vi "iterative_thinned_image_to_segment.vi"(3 "1D image array":u8[](array[numeric]), 4 "Segment Start Idx":i32, 5 "Image Height":i32) -> (0 "Algorithm timed out":bool, 1 "Endpoints":i32[](array[numeric]), 2 "Segment Sequence Cluster Arrays":cluster{i32[]}[](array[cluster]))   [LabVIEW 2019]
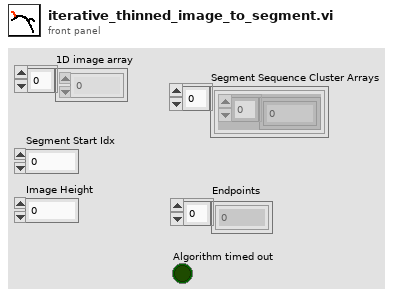
[diagram p1: front panel]
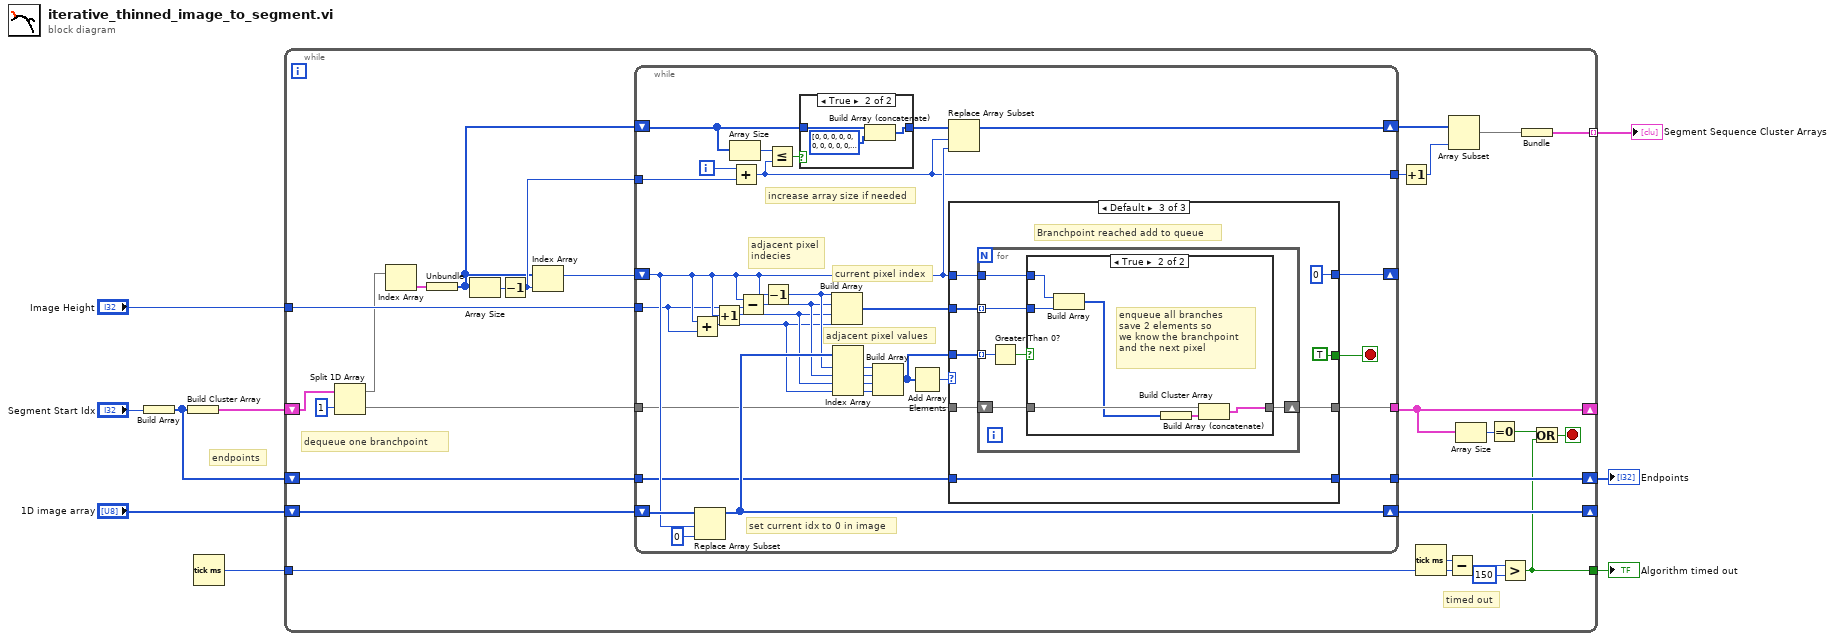
[diagram p0: block diagram]
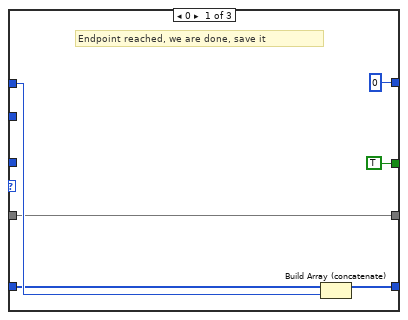
[diagram p3: hidden frame]
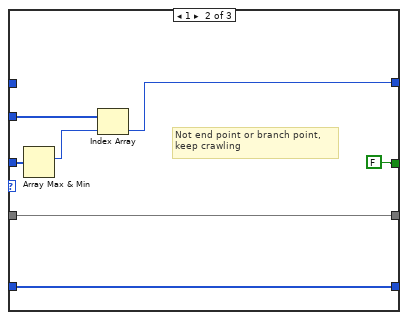
[diagram p4: hidden frame]
diagram:
  # "endpoints"
  n1 = Build Array("Segment Start Idx") -> (w4:i32[])
  n2 = Build Cluster Array(w4) -> (w3:cluster{i32[]}[])
  n3 = Tick Count (ms)() -> (millisecond timer value=w6:u32)
  n4 = while {
    shift-right: [w31] -> _
    shift-left: "1D image array" -> [w34]
    shift-right: [w24] -> _
    shift-left: w3 -> [w33]
    shift-right: [w37] -> w9
    shift-left: w4 -> [w29]
    tunnel: w6 -> [w18]
    tunnel: [w17] -> w5
    tunnel: "Image Height" -> [w16]
    tunnel: [w10] -> w1 mode=indexing
    stop <- w20 stop-if-true
    # "timed out"
    # "dequeue one branchpoint"
    n5 = Split 1D Array(array=w33, index=1 ("length")) -> (first subarray=w12:cluster{i32[]}[], second subarray=w11:cluster{i32[]}[])
    n6 = Index Array(array=w12) -> (element=w28:cluster{i32[]})  [unwired: 1 in]
    n7 = Unbundle(w28) -> (w14:i32[])
    n8 = Array Size(array=w14) -> (size(s)=w27:i32)
    n9 = Decrement(x=w27) -> (x-1=w25:i32)
    n10 = Index Array(array=w14, index=w25) -> (element=w26:i32)
    n11 = while {
      shift-right: [w38] -> w13
      shift-left: w14 -> [w39]
      shift-right: [w67] -> _
      shift-left: w26 -> [w51]
      shift-right: [w57] -> w31
      shift-left: w34 -> [w66]
      tunnel: [w52] -> w37
      tunnel: [w43] -> w36
      tunnel: w29 -> [w46]
      tunnel: w11 -> [w45]
      tunnel: [w44] -> w24
      tunnel: w25 -> [w41]
      tunnel: w16 -> [w40]
      i -> [w42]
      stop <- w47 stop-if-true
      # "current pixel index"
      # "increase array size if needed"
      # "adjacent pixel values"
      # "adjacent pixel\nindecies"
      # "set current idx to 0 in image"
      n12 = Add(x=w51, y=w40) -> (x+y=w53:i32)
      n13 = Replace Array Subset(array=w66, new element=u8 0 ("element"), index=w51) -> (w57:u8[])
      n14 = Increment(x=w51) -> (x+1=w54:i32)
      n15 = Array Size(array=w39) -> (size(s)=w50:i32)
      n16 = Add(x=w42, y=w41) -> (x+y=w43:i32)
      n17 = Subtract(x=w51, y=w40) -> (x-y=w55:i32)
      n18 = Decrement(x=w51) -> (x-1=w56:i32)
      n19 = Less Or Equal?(x=w50, y=w43) -> (x <= y?=w49:bool)
      n20 = case shown="True" w49 {
        tunnel: w39 -> [w68 w71]
        tunnel: [w68 w70] -> w48
        frame False {
        }
        frame True {
          n21 = Build Array (concatenate)(w71, i32[] [0, 0, 0, 0, 0, 0, 0, 0, 0, 0, 0, 0, 0, 0, 0, 0, 0, 0, 0, 0, 0, 0, 0, 0, 0, 0, 0, 0, 0, 0, 0] ("array")) -> (w70:i32[])
        }
      }
      n22 = Build Array(w56, w55, w54, w53) -> (w58:i32[])
      n23 = Index Array(array=w57, index #1=w56, index #2=w55, index #3=w54, index #4=w53) -> (element #1=w63:u8, element #2=w62:u8, element #3=w61:u8, element #4=w60:u8)
      n24 = Build Array(w63, w62, w61, w60) -> (w59:u8[])
      n25 = Add Array Elements(numeric array=w59) -> (sum=w64:u8)
      n26 = Replace Array Subset(array=w48, new element=w51, index=w43) -> (w38:i32[])
      n27 = case shown="Default" w64 {
        tunnel: [TRUE FALSE TRUE] -> w47
        tunnel: [0 w80 0] -> w67
        tunnel: w59 -> [_ w83 w90]
        tunnel: w58 -> [_ w82 w89]
        tunnel: w51 -> [w75 _ w85]
        tunnel: [w74 w79 w91] -> w52
        tunnel: w46 -> [w73 w79 w91]
        tunnel: w45 -> [w72 w78 w88]
        tunnel: [w72 w78 w86] -> w44
        frame 0 {
          # "Endpoint reached, we are done, save it"
          n28 = Build Array (concatenate)(w73, w75) -> (w74:i32[])
        }
        frame 1 {
          # "Not end point or branch point,\nkeep crawling"
          n29 = Array Max & Min(array=w83) -> (max index (indices)=w81:i32)  [unwired: 3 out]
          n30 = Index Array(array=w82, index=w81) -> (element=w80:i32)
        }
        frame Default {
          # "Branchpoint reached add to queue"
          n31 = for {
            tunnel: w90 -> [w98] mode=indexing
            tunnel: w89 -> [w96] mode=indexing
            shift-right: [w94] -> w86
            shift-left: w88 -> [w95]
            tunnel: w85 -> [w93]
            n32 = Greater Than 0?(x=w98) -> (x > 0?=w97:bool)
            n33 = case shown="True" w97 {
              tunnel: w96 -> [_ w102]
              tunnel: w95 -> [w99 w105]
              tunnel: [w99 w104] -> w94
              tunnel: w93 -> [_ w103]
              frame False {
                # "not a branch"
              }
              frame True {
                # "enqueue all branches\nsave 2 elements so\nwe know the branchpoint\nand the next pixel"
                n34 = Build Array(w103, w102) -> (w101:i32[])
                n35 = Build Cluster Array(w101) -> (w100:cluster{i32[]}[])
                n36 = Build Array (concatenate)(w105, w100) -> (w104:cluster{i32[]}[])
              }
            }
          }
        }
      }
    }
    n37 = Increment(x=w36) -> (x+1=w15:i32)
    n38 = Tick Count (ms)() -> (millisecond timer value=w23:u32)
    n39 = Subtract(x=w23, y=w18) -> (x-y=w22:u32)
    n40 = Array Subset(array=w13, length=w15) -> (w35:i32[])  [unwired: 1 in]
    n41 = Array Size(array=w24) -> (size(s)=w30:i32)
    n42 = Equal To 0?(x=w30) -> (x = 0?=w19:bool)
    n43 = Greater?(x=w22, y=u32 150) -> (0:w17:bool)
    n44 = Bundle(w35) -> (w10:cluster{i32[]})  [unwired: 1 in]
    n45 = Or(x=w19, y=w17) -> (x .or. y?=w20:bool)
  }
  "Endpoints" <- w9
  "Algorithm timed out" <- w5
  "Segment Sequence Cluster Arrays" <- w1
